vi "Start Logger.vi"(8 "error in (no error)":errorcluster, 9 "Do not store ref":bool, 11 "Monitor Controller in":refnum<class "Monitor Controller.lvclass">) -> (0 "error out":errorcluster, 1 "tdms ref out":refnum<k34>, 2 "File Path":path, 3 "Monitor Controller out":refnum<class "Monitor Controller.lvclass">)   [LabVIEW 2016, in "Monitor Controller.lvclass"]
uses:
  Monitor Controller.lvclass
  Measure_extentions/Monitor-Pulse Messages/Write Monitor File Msg/Write Monitor File Msg.lvclass
  <vilib>/ActorFramework/Actor/Actor.lvclass
  Process Controller/Process Controller.lvclass
  Measure_extentions/Monitor-Pulse Messages/Update Monitor State Msg/Update Monitor State Msg.lvclass
  C:/Program Files/National Instruments/LabVIEW 2016/vi.lib/ActorFramework/Actor/Actor.lvclass
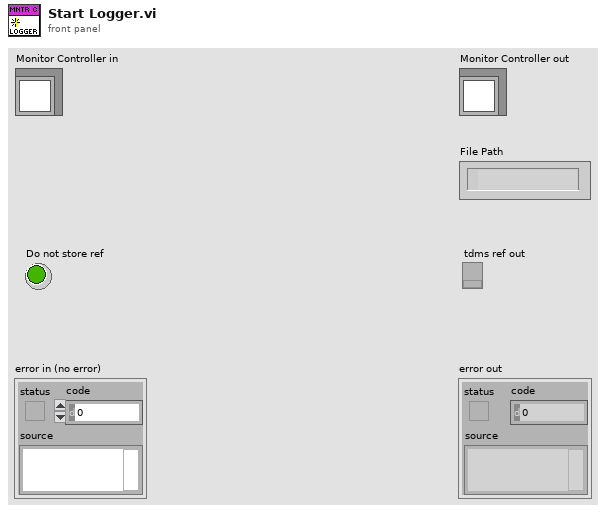
[diagram p1: front panel]
types:
  T1 = typedef "Monitor Controller Configuration.ctl" = cluster{"Update period":dbl, "Repeat times":i32, "Open plot":bool, "File defragment period":dbl}
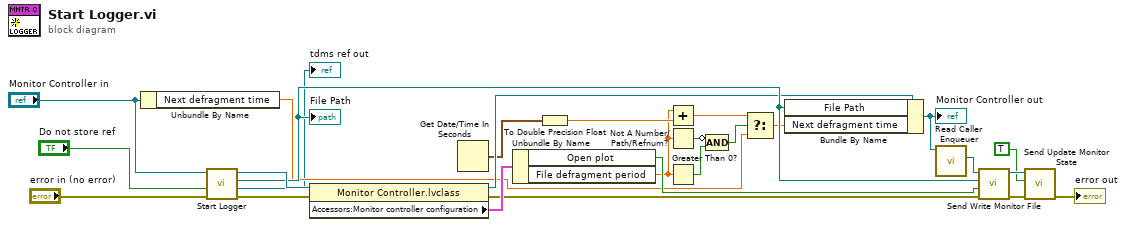
[diagram p0: block diagram]
diagram:
  n1 = Unbundle By Name("Monitor Controller in") -> ("Next defragment time"=w7:dbl)
  n2 = call-parent "Start Logger.vi"("error in (no error)"="error in (no error)", "Do not store ref"="Do not store ref", "Measure Controller in"="Monitor Controller in") -> ("error out"=w18:errorcluster, "tdms ref out"=→"tdms ref out":refnum<k34>, "File Path"=w22:path, "Measure Controller out"=w25:refnum<class "Monitor Controller.lvclass">)  [unwired: 5 in]
  "File Path" <- w22
  n3 = property class="Monitor Controller.lvclass"(reference=w25, error in=w18) -> (reference out=w21:refnum<class "Monitor Controller.lvclass">, error out=w17:errorcluster, "Accessors:Monitor controller configuration"=w20:T1)
  n4 = Get Date/Time In Seconds() -> (seconds since 1Jan1904=w14:timestamp)
  n5 = Unbundle By Name(w20) -> ("Open plot"=w19:bool, "File defragment period"=w12:dbl)
  n6 = To Double Precision Float(number=w14) -> (double precision float=w13:dbl)
  n7 = Add(x=w12, y=w13) -> (x+y=w9:dbl)
  n8 = Not A Number/Path/Refnum?(number/path/refnum=w12) -> (NaN/Path/Refnum?=w16:bool)
  n9 = Greater Than 0?(x=w12) -> (x > 0?=w15:bool)
  n10 = Compound Arithmetic op=AND(invert w16, w15) -> (w10:bool)
  n11 = Select(t=w9, s=w10, f=w7) -> (s? t:f=w8:dbl)
  n12 = Bundle By Name(cluster=w21, "File Path"=w22, "Next defragment time"=w8) -> (w23:refnum<class "Monitor Controller.lvclass">)
  "Monitor Controller out" <- w23
  n13 = call <vilib>:"Read Caller Enqueuer.vi"("Actor"=w23) -> ("Caller Enqueuer"=w24:refnum<class "Message Enqueuer.lvclass">)  [unwired: 10 in]
  n14 = call "Send Write Monitor File.vi"("error in (no error)"=w17, "Open plot"=w19, "Monitor File"=w22, "Message Enqueuer"=w24) -> ("error out"=w6:errorcluster, "Message Enqueuer out"=w5:refnum<class "Message Enqueuer.lvclass">)  [unwired: 6 in]
  n15 = call "Send Update Monitor State.vi"("error in (no error)"=w6, "Monitor Running"=TRUE, "Message Enqueuer"=w5) -> ("error out"=→"error out":errorcluster)  [unwired: 7 in, 1 out]
